vi "存储.vi"() -> ()   [LabVIEW 2018]
uses:
  <vilib>/Utility/file.llb/Write Delimited Spreadsheet (string).vi
panel:
  in  "file path (dialog if empty)":path caption="文件路径 （空时为对话框）"
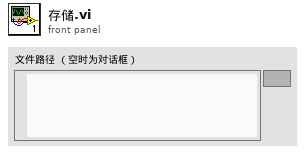
[diagram p1: front panel]
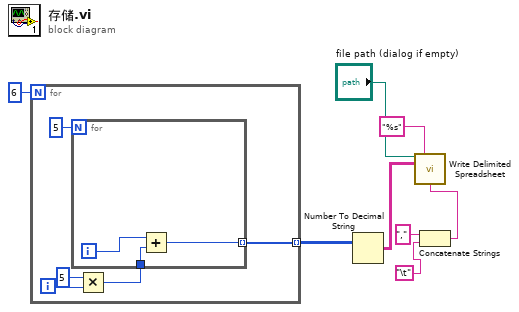
[diagram p0: block diagram]
diagram:
  n1 = for {
    N: 6 -> [_]
    tunnel: [w9] -> w5 mode=indexing
    i -> [w12]
    n2 = Multiply(x=5, y=w12) -> (x*y=w10:i32)
    n3 = for {
      N: 5 -> [_]
      tunnel: w10 -> [w16]
      tunnel: [w14] -> w9 mode=indexing
      i -> [w15]
      n4 = Add(x=w15, y=w16) -> (x+y=w14:i32)
    }
  }
  n5 = Number To Decimal String(number=w5) -> (decimal integer string=w4:string[][])  [unwired: 1 in]
  n6 = Concatenate Strings("," ("字符串"), "\t") -> (w1:string)
  n7 = call-poly <vilib>:"Write Delimited Spreadsheet.vi"("file path (dialog if empty)"="file path (dialog if empty)", "format (%s)"="%s" ("format (%d)"), "2D data"=w4, "delimiter (\\t)"=w1) -> ()  [unwired: 10 in, 2 out]
